vi "Revision Query.vi"(8 "error in (no error)":errorcluster, 11 "CS++DCPwr in":refnum<class "CS++DCPwr.lvclass">) -> (0 "error out":errorcluster, 1 "Firmware Revision":string, 2 "Driver Revision":string, 3 "CS++DCPwr out":refnum<class "CS++DCPwr.lvclass">)   [LabVIEW 2013, in "CS++DCPwr.lvlib" / "CS++DCPwr.lvclass"]
uses:
  CS++DCPwr.lvclass
  Core/Actors/CS++DeviceActor/CS++DeviceActor.lvclass
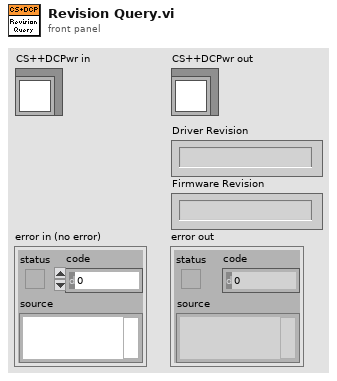
[diagram p1: front panel]
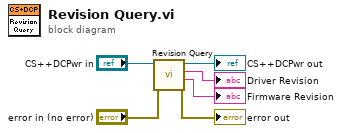
[diagram p0: block diagram]
diagram:
  n1 = call-parent "Revision Query.vi"("error in (no error)"="error in (no error)", "CS++DeviceActor in"="CS++DCPwr in") -> ("error out"=→"error out":errorcluster, "Firmware Revision"=→"Firmware Revision":string, "Driver Revision"=→"Driver Revision":string, "CS++DeviceActor out"=→"CS++DCPwr out":refnum<class "CS++DCPwr.lvclass">)  [unwired: 6 in]
